vi "Write PS Driver.vi"(8 "error in (no error)":errorcluster, 10 "PS Driver.lvlib:PS Driver.lvclass":refnum<class "PS Driver.lvclass">, 11 "PS Control Actor in":refnum<class "PS Control Actor.lvclass">) -> (0 "error out":errorcluster, 3 "PS Control Actor out":refnum<class "PS Control Actor.lvclass">)   [LabVIEW 2019, in "PS Control Actor.lvlib" / "PS Control Actor.lvclass"]
uses:
  PS Control Actor.lvclass
  PS Driver/PS Driver.lvclass
  PS Control Actor.lvclass/PS Control Actor.ctl
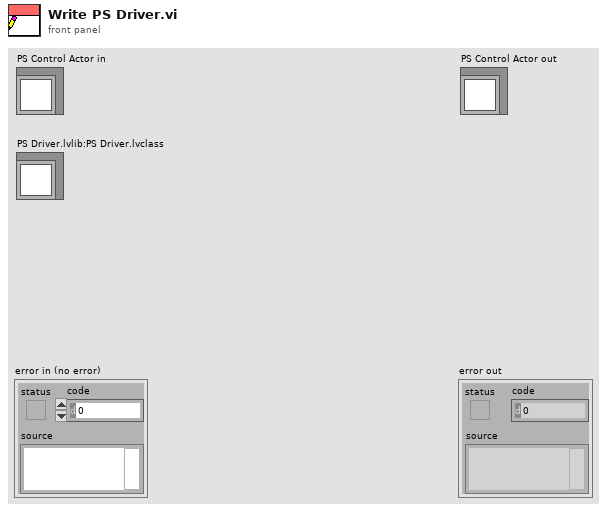
[diagram p1: front panel]
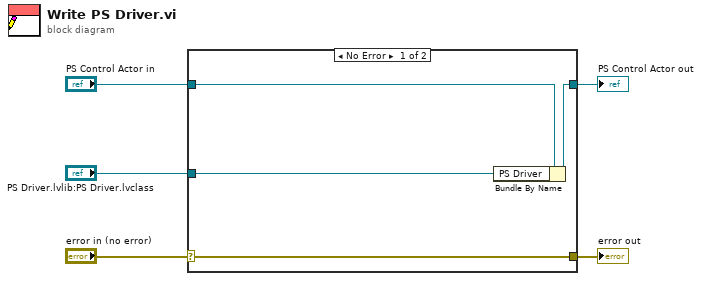
[diagram p0: block diagram]
diagram:
  n1 = case shown="No Error" "error in (no error)" {
    selector: "error in (no error)" -> [w9 w10]
    tunnel: [w9 w10] -> w4
    tunnel: [w7 w11] -> w2
    tunnel: "PS Control Actor in" -> [w8 w11]
    tunnel: "PS Driver.lvlib:PS Driver.lvclass" -> [w6 _]
    frame No Error {
      n2 = Bundle By Name(cluster=w8, "PS Driver"=w6) -> (w7:refnum<class "PS Control Actor.lvclass">)
    }
    frame Error {
    }
  }
  "error out" <- w4
  "PS Control Actor out" <- w2
